vi "Versa Planet.vi"(7 "Description":string, 11 "Setpoint":dbl) -> ()   [LabVIEW 2015]
uses:
  <vilib>/Rock Robotics/WPI/Framework/Command Status Info.ctl
  <vilib>/Rock Robotics/WPI/Framework/Completion Status.ctl
  <vilib>/Rock Robotics/WPI/Framework/Completion Notifier.ctl
  Implementation/Test Setpoints.ctl
  Implementation/Test Operations.ctl
panel:
  out "Command Info Out":T1
  in  "Command Info In":T1
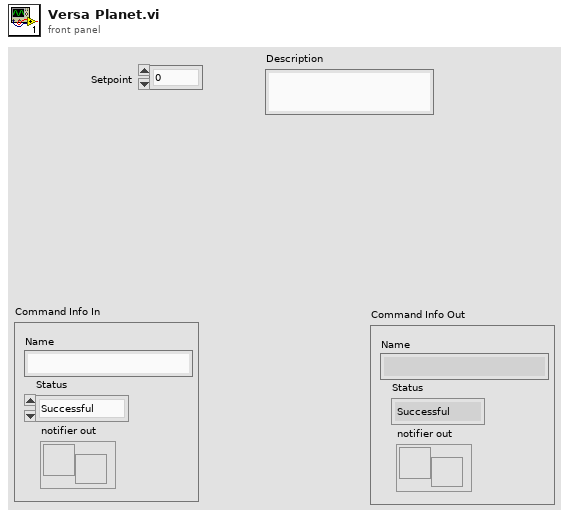
[diagram p1: front panel]
types:
  T1 = typedef "Command Status Info.ctl" = cluster{"Name":string, "Status":T2, "notifier out":T3}
  T2 = typedef "Completion Status.ctl" = enum16{"Successful", "Aborted", "Incomplete"}
  T3 = typedef "Completion Notifier.ctl" = refnum<notifier>
  T4 = typedef "Test Setpoints.ctl" = cluster{"Operation":T5, "Setpoint":dbl, "Duration":dbl}
  T5 = typedef "Test Operations.ctl" = enum16{"Reserve", "Read Current", "Immediate", "Test PID Motor"}
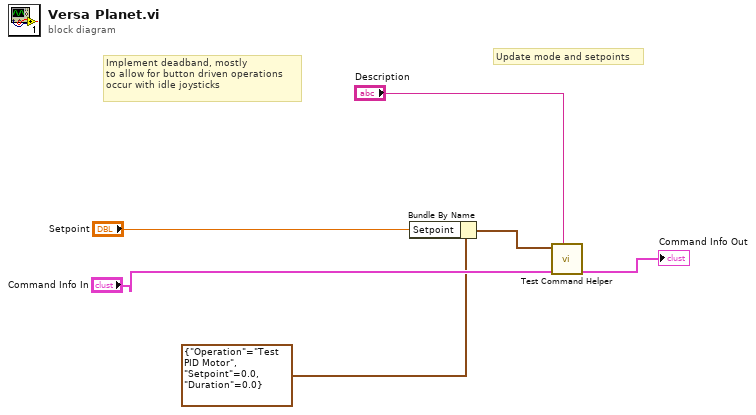
[diagram p0: block diagram]
diagram:
  # "Implement deadband, mostly\nto allow for button driven operations\noccur with idle joysticks"
  # "Update mode and setpoints"
  n1 = Bundle By Name(cluster=T4 {"Operation"=enum."Test PID Motor", "Setpoint"=0.0, "Duration"=0.0} ("SubSystem Data"), "Setpoint"="Setpoint") -> (w3:T4)
  n2 = call "Test Command Helper.vi"("Description"="Description", "Command Info In"="Command Info In", "SubSystem Data"=w3) -> ("Command Info Out"=→"Command Info Out":T1)  [unwired: 7 in, 1 out]
